vi "4.6.2.vi"() -> ()   [LabVIEW 2017]
panel:
  in  "stop止":bool
  out "和":dbl
  in  "b":dbl
  in  "a":dbl
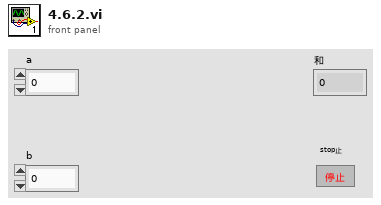
[diagram p1: front panel]
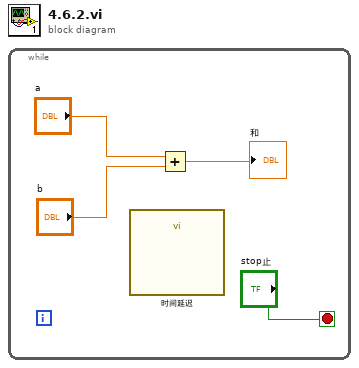
[diagram p0: block diagram]
diagram:
  n1 = while {
    stop <- "stop止" stop-if-true
    n2 = call "时间延迟"() -> ()  [unwired: 11 in, 1 out]
    n3 = Add(x="a", y="b") -> (x+y=→"和":dbl)
  }
